vi "Send datagram over udp.vi"(7 "Data":u32[](array[numeric]) format="%.0x", 8 "error in (no error)":errorcluster, 9 "port":u16, 10 "Address":u32, 11 "IDP ref":refnum<k16>) -> (0 "error out":errorcluster)   [LabVIEW 2015]
panel:
  out "size(s)":i32
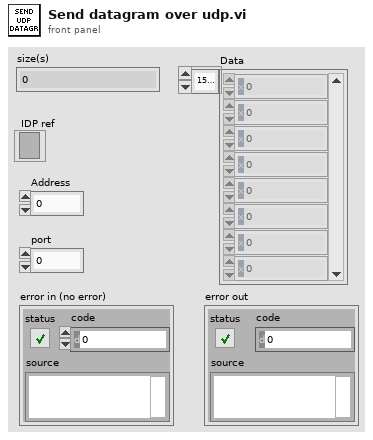
[diagram p1: front panel]
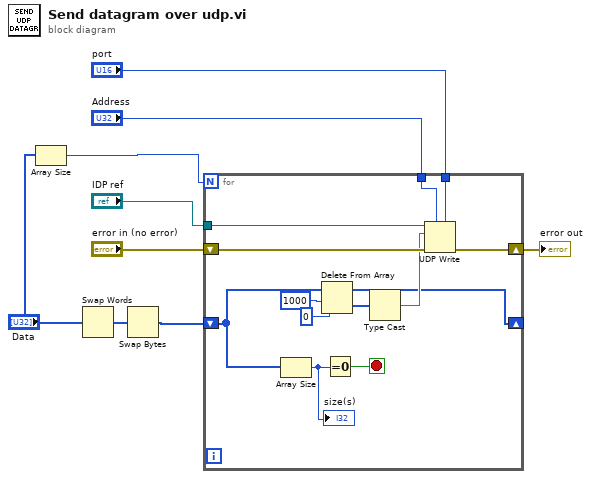
[diagram p0: block diagram]
diagram:
  n1 = Array Size(array="Data") -> (size(s)=w4:i32)
  n2 = Swap Words(1:"Data") -> (0:w2:u32[])
  n3 = Swap Bytes(anything=w2) -> (byte swapped=w1:u32[])
  n4 = for {
    N: w4 -> [_]
    tunnel: "port" -> [w20]
    tunnel: "IDP ref" -> [w19]
    tunnel: "Address" -> [w18]
    shift-right: [w22] -> w9
    shift-left: "error in (no error)" -> [w21]
    shift-right: [w11] -> _
    shift-left: w1 -> [w15]
    stop <- w16 stop-if-true
    n5 = Array Size(array=w15) -> (size(s)=w17:i32)
    "size(s)" <- w17
    n6 = Delete From Array(array=w15, length=1000, index=0) -> (deleted portion=w13:u32[], array with subset deleted=w11:u32[])
    n7 = Equal To 0?(x=w17) -> (x = 0?=w16:bool)
    n8 = Type Cast(x=w13) -> (*(type *) &x=w12:string)  [unwired: 1 in]
    n9 = UDP Write(address=w18, port or service name=w20, connection ID=w19, data in=w12, 8:w21) -> (error out=w22:errorcluster)  [unwired: 1 in, 1 out]
  }
  "error out" <- w9
